vi "SHAPE_GA_Create Population.vi"(5 "Function Data":variant, 6 "Parameters":T2={"Population size"=100, "Generations no."=500, "Significant digits"=4, "Crossover probabality"=0.85, "Mutation mode"=enum."one-point, fixed rate", "Use Gray code?"=FALSE, "Mutation rate"=0.05, "Min mutation rate"=0.0005, "Max mutation rate"=0.25, "Reproduction plan"=enum."Steady-state-replace-worst", "Elitism"=FALSE, "Fmax"=1} {"Max mutation rate" min=0.0 max=1.0; "Min mutation rate" min=0.0 max=1.0; "Mutation rate" min=0.0 max=1.0; "Crossover probabality" min=0.0 max=1.0; "Significant digits" min=1; "Generations no." min=1; "Population size" min=1}, 7 "Fitness Function":T3, 8 "Phenotype size":i32, 9 "Population size":i32) -> (3 "Population out":T1)   [LabVIEW 2016, in "Shapelets Search (GA).lvlib"]
doc: "Randomizes population and calculate fitnesses"
uses:
  Shapelets Search (GA).lvlib
  5. Features Optimization/_Optimal Frequency Bands Search/GA_core/GA_tFitness Function.ctl
  5. Features Optimization/_Optimal Frequency Bands Search/GA_core/GA_tParameters.ctl
  5. Features Optimization/_Optimal Frequency Bands Search/GA_core/GA_tPopulation.ctl
  <vilib>/gmath/statdist.llb/Uniform (Discrete) Random.vi
  <vilib>/gmath/NI_Gmath.lvlib
  5. Features Optimization/_Optimal Frequency Bands Search/GA_core/GeneticAlgorithm.lvlib
panel:
  # "This VI is a part of BCI Design library, http://www.ru-bci.org \nCopyright © 2020, Sotnikov Peter, All rights reserved. License: CC BY-NC 4.0"
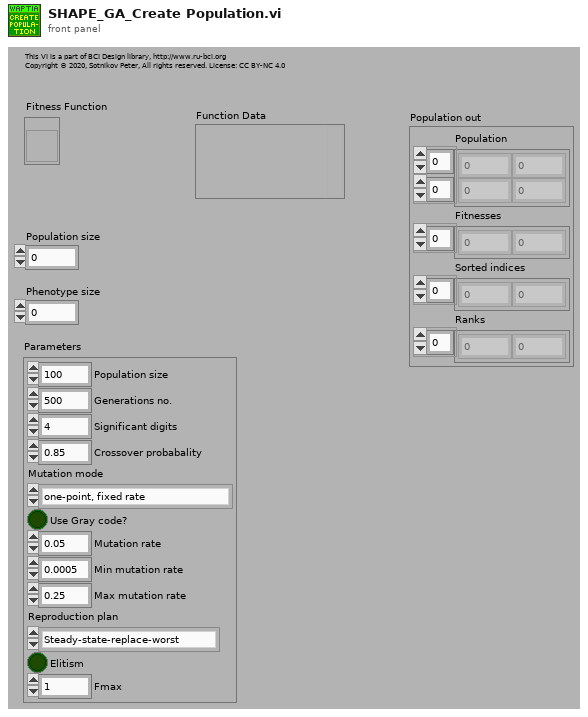
[diagram p1: front panel]
types:
  T1 = typedef "Optimal Frequency Bands Search.lvlib/GeneticAlgorithm.lvlib/GA_tPopulation.ctl" = cluster{"Population":i32[][], "Fitnesses":dbl[], "Sorted indices":i32[], "Ranks":i32[]}
  T2 = typedef "Optimal Frequency Bands Search.lvlib/GeneticAlgorithm.lvlib/GA_tParameters.ctl" = cluster{"Population size":i32, "Generations no.":i32, "Significant digits":i32, "Crossover probabality":dbl, "Mutation mode":enum16{"one-point, fixed rate", "one-point, fitness-adjustable rate", "one-point, distance-adjustable rate"}, "Use Gray code?":bool, "Mutation rate":dbl, "Min mutation rate":dbl, "Max mutation rate":dbl, "Reproduction plan":enum16{"Full generational replacement", "Steady-state-replace-random", "Steady-state-replace-worst"}, "Elitism":bool, "Fmax":i32}
  T3 = typedef "Optimal Frequency Bands Search.lvlib/GeneticAlgorithm.lvlib/GA_tFitness Function.ctl" = refnum<vi>
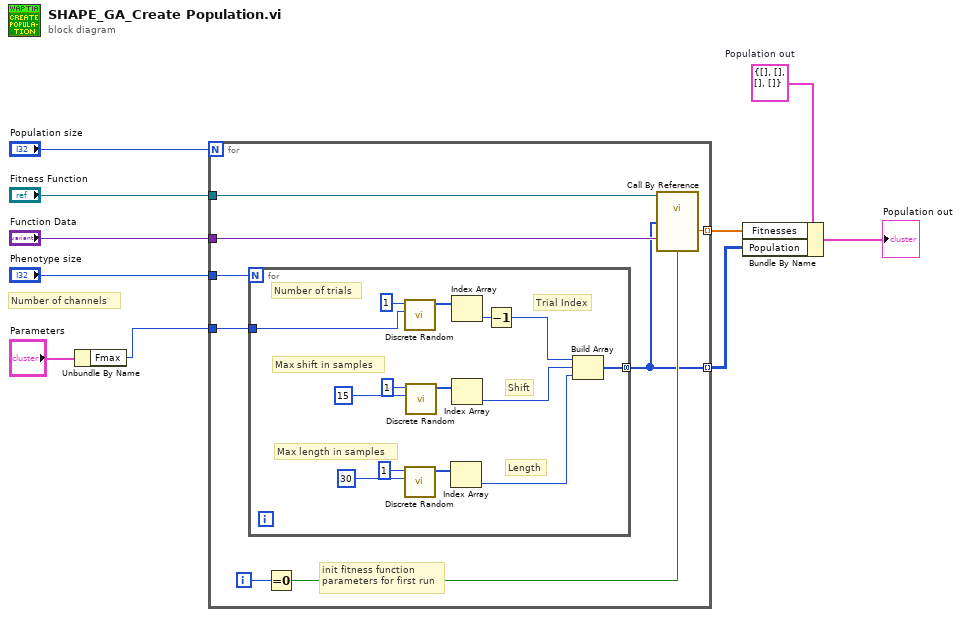
[diagram p0: block diagram]
diagram:
  w7 = T1 {"Population"=[], "Fitnesses"=[], "Sorted indices"=[], "Ranks"=[]}  # Population out
  # "Number of channels"
  n1 = Unbundle By Name("Parameters") -> ("Fmax"=w1:i32)
  n2 = for {
    N: "Population size" -> [_]
    tunnel: "Phenotype size" -> [w12]
    tunnel: "Fitness Function" -> [w16]
    tunnel: [w18] -> w6 mode=indexing
    tunnel: [w13] -> w5 mode=indexing
    tunnel: "Function Data" -> [w17]
    tunnel: w1 -> [w11]
    i -> [w15]
    # "init fitness function\nparameters for first run"
    n3 = for {
      N: w12 -> [_]
      tunnel: [w30] -> w13 mode=concatenating
      tunnel: w11 -> [w19]
      # "Max length in samples"
      # "Max shift in samples"
      # "Number of trials"
      # "Length"
      # "Shift"
      # "Trial Index"
      n4 = call-poly <vilib>:"Discrete Random.vi"("n"=w19, "samples"=1) -> ("uniform (discrete) random data"=w28:i32[])  [unwired: 8 in, 1 out]
      n5 = call-poly <vilib>:"Discrete Random.vi"("n"=30, "samples"=1) -> ("uniform (discrete) random data"=w21:i32[])  [unwired: 8 in, 1 out]
      n6 = call-poly <vilib>:"Discrete Random.vi"("n"=15, "samples"=1) -> ("uniform (discrete) random data"=w24:i32[])  [unwired: 8 in, 1 out]
      n7 = Index Array(array=w21) -> (element=w20:i32)  [unwired: 1 in]
      n8 = Index Array(array=w28) -> (element=w27:i32)  [unwired: 1 in]
      n9 = Index Array(array=w24) -> (element=w31:i32)  [unwired: 1 in]
      n10 = Decrement(x=w27) -> (x-1=w32:i32)
      n11 = Build Array(w32, w31, w20) -> (w30:i32[])
    }
    n12 = Equal To 0?(x=w15) -> (x = 0?=w14:bool)
    n13 = call-by-ref "?"(reference=w16, "Init? (F)"=w14, "Data"=w17, "Phenotype"=w13) -> ("Fitness"=w18:dbl)  [unwired: 1 in, 2 out]
  }
  n14 = Bundle By Name(cluster=w7, "Fitnesses"=w6, "Population"=w5) -> (→"Population out":T1)
